vi "PXI-DO Signal Bank.vi"(7 "Array":bool[][](array[boolean]), 11 "error in (no error)":errorcluster, 13 "Action":T1) -> (8 "Array out":bool[][](array[boolean]), 15 "error out":errorcluster)   [LabVIEW 2020]
uses:
  Type Defs/PXI-DO Signal Bank Action.ctl
  DAQ Engine VIs/PXI Globals.vi
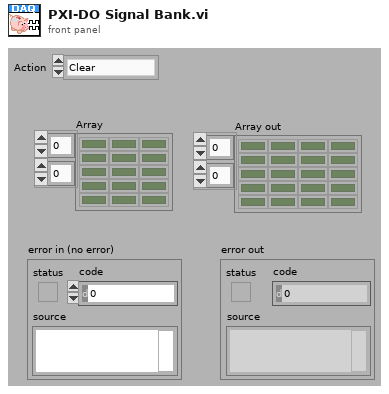
[diagram p1: front panel]
types:
  T1 = typedef "PXI-DO Signal Bank Action.ctl" = enum16{"Clear", "Write", "Read"}
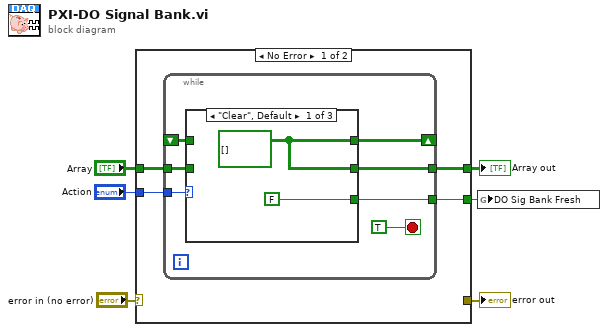
[diagram p0: block diagram]
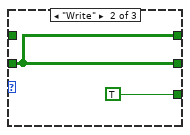
[diagram p2: hidden frame]
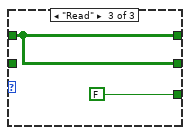
[diagram p3: hidden frame]
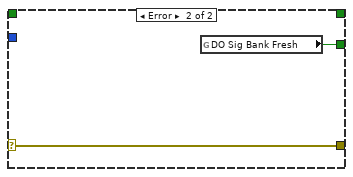
[diagram p4: hidden frame]
diagram:
  n1 = case shown="No Error" "error in (no error)" {
    selector: "error in (no error)" -> [_ w25]
    tunnel: "Action" -> [w10 _]
    tunnel: "Array" -> [w9 _]
    tunnel: [w8 _] -> w1
    tunnel: [w7 w24] -> w4
    tunnel: [_ w25] -> w2
    frame No Error {
      n2 = while {
        tunnel: w10 -> [w16]
        shift-right: [w15] -> _
        shift-left: _ -> [w14]
        tunnel: w9 -> [w13]
        tunnel: [w12] -> w8
        tunnel: [w11] -> w7
        stop <- TRUE stop-if-true
        n3 = case shown="\"Clear\", Default" w16 {
          tunnel: [w19 w20 w23] -> w15
          tunnel: w14 -> [_ _ w23]
          tunnel: w13 -> [_ w20 _]
          tunnel: [w19 w20 w23] -> w12
          tunnel: [FALSE ("DO Sig Bank Read") TRUE ("DO Sig Bank Read") FALSE ("DO Sig Bank Read")] -> w11
          frame "Clear", Default {
            w19 = bool[][] []
          }
          frame "Write" {
          }
          frame "Read" {
          }
        }
      }
    }
    frame Error {
      n4 = global read "PXI Globals.vi" "DO Sig Bank Fresh"() -> (w24:bool)
    }
  }
  "Array out" <- w1
  "error out" <- w2
  n5 = global write "PXI Globals.vi" "DO Sig Bank Fresh"(w4) -> ()
